vi "CNC-SpikePrime.vi"() -> ()   [LabVIEW 2020]
uses:
  Subs/ColorText/Code.xctl
panel:
  out "Array":dbl[][](array[numeric]) format="%#.2f"
  out "Bounds":T1 {"F Max" format="%#.1f"; "F Min" format="%#.1f"; "Z Max" format="%#.1f"; "Z Min" format="%#.1f"; "Y Max" format="%#.1f"; "Y Min" format="%#.1f"; "X Max" format="%#.1f"; "X Min" format="%#.1f"}
  out "Code":string(xcontrol)="import os\n\nfor i in range(10):\n     print(i)\n"
  in  "file (use dialog)":path=path "/Users/crogers/Downloads/PiMount_2.gcode"
  out "text":string="$X\nG21\nG90\nM6 T1\nG0 Z1.0 F300\nG0 X82.55 Y117.475 F6000\nG1 Z-2.2758 F250\nG1 Y123.825 F1000\nG1 X171.45\nG1 Y117.475\nG1 X82.55\nG1 X79.375 Y114.3\nG1 Y127.0\nG1 X174.625\nG1 Y114.3\nG1 X79.375\nG1 X76.2 Y111.125\nG1 Y130.175\nG1 X177.8\nG1 Y111.125\nG1 X76.2\nG1 X73.025 Y107.95\nG1 Y133.35\nG1 X180.975\nG1 Y107.95\nG1 X73.025\nG1 X69.85 Y104.775\nG1 Y136.525\nG1 X184.15\nG1 Y104.775\nG1 X69.85\nG1 X66.675 Y101.6\nG1 Y139.7\nG1 X187.325\nG1 Y101.6\nG1 X66.675\nG1 X63.5 Y98.425\nG1 Y142.875\nG1 X190.5\nG1 Y98.425\nG1 X63.5\nG1 X60.325 Y95.25\nG1 Y146.05\nG1 X193.675\nG1 Y95.25\nG1 X60.325\nG1 X57.15 Y92.075\nG1 Y149.225\nG1 X196.85\nG1 Y92.075\nG1 X57.15\nG1 X53.975 Y88.9\nG1 Y152.4\nG1 X200.025\nG1 Y88.9\nG1 X53.975\nG1 X50.8 Y85.725\nG1 Y155.575\nG1 X203.2\nG1 Y85.725\nG1 X50.8\nG1 X47.625 Y82.55\nG1 Y158.75\nG1 X206.375\nG1 Y82.55\nG1 X47.625\nG1 X44.45 Y79.375\nG1 Y161.925\nG1 X209.55\nG1 Y79.375\nG1 X44.45\nG1 X41.275 Y76.2\nG1 Y165.1\nG1 X212.725\nG1 Y76.2\nG1 X41.275\nG1 X38.1 Y73.025\nG1 Y168.275\nG1 X215.9\nG1 Y73.025\nG1 X38.1\nG1 X34.925 Y69.85\nG1 Y171.45\nG1 X219.075\nG1 Y69.85\nG1 X34.925\nG1 X31.8279 Y66.675\nG1 X31.7536 Y66.6787\nG1 X31.75 Y66.7528\nG1 Y174.5472\nG1 X31.7536 Y174.6214\nG1 X31.8279 Y174.625\nG1 X222.1721\nG1 X222.2464 Y174.6214\nG1 X222.25 Y174.5472\nG1 Y66.7528\nG1 X222.2464 Y66.6787\nG1 X222.1721 Y66.675\nG1 X31.8279\nG0 Z1.0 F300\nG0 X82.55 Y117.475 F6000\nG1 Z-4.2113 F250\nG1 Y123.825 F1000\nG1 X171.45\nG1 Y117.475\nG1 X82.55\nG1 X79.375 Y114.3\nG1 Y127.0\nG1 X174.625\nG1 Y114.3\nG1 X79.375\nG1 X76.2 Y111.125\nG1 Y130.175\nG1 X177.8\nG1 Y111.125\nG1 X76.2\nG1 X73.025 Y107.95\nG1 Y133.35\nG1 X180.975\nG1 Y107.95\nG1 X73.025\nG1 X69.85 Y104.775\nG1 Y136.525\nG1 X184.15\nG1 Y104.775\nG1 X69.85\nG1 X66.675 Y101.6\nG1 Y139.7\nG1 X187.325\nG1 Y101.6\nG1 X66.675\nG1 X63.5 Y98.425\nG1 Y142.875\nG1 X190.5\nG1 Y98.425\nG1 X63.5\nG1 X60.325 Y95.25\nG1 Y146.05\nG1 X193.675\nG1 Y95.25\nG1 X60.325\nG1 X57.15 Y92.075\nG1 Y149.225\nG1 X196.85\nG1 Y92.075\nG1 X57.15\nG1 X53.975 Y88.9\nG1 Y152.4\nG1 X200.025\nG1 Y88.9\nG1 X53.975\nG1 X50.8 Y85.725\nG1 Y155.575\nG1 X203.2\nG1 Y85.725\nG1 X50.8\nG1 X47.625 Y82.55\nG1 Y158.75\nG1 X206.375\nG1 Y82.55\nG1 X47.625\nG1 X44.45 Y79.375\nG1 Y161.925\nG1 X209.55\nG1 Y79.375\nG1 X44.45\nG1 X41.275 Y76.2\nG1 Y165.1\nG1 X212.725\nG1 Y76.2\nG1 X41.275\nG1 X38.1 Y73.025\nG1 Y168.275\nG1 X215.9\nG1 Y73.025\nG1 X38.1\nG1 X34.925 Y69.85\nG1 Y171.45\nG1 X219.075\nG1 Y69.85\nG1 X34.925\nG1 X31.8279 Y66.675\nG1 X31.7536 Y66.6787\nG1 X31.75 Y66.7528\nG1 Y174.5472\nG1 X31.7536 Y174.6214\nG1 X31.8279 Y174.625\nG1 X222.1721\nG1 X222.2464 Y174.6214\nG1 X222.25 Y174.5472\nG1 Y66.7528\nG1 X222.2464 Y66.6787\nG1 X222.1721 Y66.675\nG1 X31.8279\nG0 Z1.0 F300\nG0 X82.55 Y117.475 F6000\nG1 Z-6.35 F250\nG1 Y123.825 F1000\nG1 X171.45\nG1 Y117.475\nG1 X82.55\nG1 X79.375 Y114.3\nG1 Y127.0\nG1 X174.625\nG1 Y114.3\nG1 X79.375\nG1 X76.2 Y111.125\nG1 Y130.175\nG1 X177.8\nG1 Y111.125\nG1 X76.2\nG1 X73.025 Y107.95\nG1 Y133.35\nG1 X180.975\nG1 Y107.95\nG1 X73.025\nG1 X69.85 Y104.775\nG1 Y136.525\nG1 X184.15\nG1 Y104.775\nG1 X69.85\nG1 X66.675 Y101.6\nG1 Y139.7\nG1 X187.325\nG1 Y101.6\nG1 X66.675\nG1 X63.5 Y98.425\nG1 Y142.875\nG1 X190.5\nG1 Y98.425\nG1 X63.5\nG1 X60.325 Y95.25\nG1 Y146.05\nG1 X193.675\nG1 Y95.25\nG1 X60.325\nG1 X57.15 Y92.075\nG1 Y149.225\nG1 X196.85\nG1 Y92.075\nG1 X57.15\nG1 X53.975 Y88.9\nG1 Y152.4\nG1 X200.025\nG1 Y88.9\nG1 X53.975\nG1 X50.8 Y85.725\nG1 Y155.575\nG1 X203.2\nG1 Y85.725\nG1 X50.8\nG1 X47.625 Y82.55\nG1 Y158.75\nG1 X206.375\nG1 Y82.55\nG1 X47.625\nG1 X44.45 Y79.375\nG1 Y161.925\nG1 X209.55\nG1 Y79.375\nG1 X44.45\nG1 X41.275 Y76.2\nG1 Y165.1\nG1 X212.725\nG1 Y76.2\nG1 X41.275\nG1 X38.1 Y73.025\nG1 Y168.275\nG1 X215.9\nG1 Y73.025\nG1 X38.1\nG1 X34.925 Y69.85\nG1 Y171.45\nG1 X219.075\nG1 Y69.85\nG1 X34.925\nG1 X31.8279 Y66.675\nG1 X31.7536 Y66.6787\nG1 X31.75 Y66.7528\nG1 Y174.5472\nG1 X31.7536 Y174.6214\nG1 X31.8279 Y174.625\nG1 X222.1721\nG1 X222.2464 Y174.6214\nG1 X222.25 Y174.5472\nG1 Y66.7528\nG1 X222.2464 Y66.6787\nG1 X222.1721 Y66.675\nG1 X31.8279\nG0 Z1.0 F300\nG0 X104.775 Y117.475 F6000\nG1 Z-8.0823 F250\nG1 Y123.825 F1000\nG1 X149.225\nG1 Y117.475\nG1 X104.775\nG1 X101.6 Y114.3\nG1 Y127.0\nG1 X152.4\nG1 Y114.3\nG1 X101.6\nG1 X98.425 Y111.125\nG1 Y130.175\nG1 X155.575\nG1 Y111.125\nG1 X98.425\nG1 X95.25 Y107.95\nG1 Y133.35\nG1 X158.75\nG1 Y107.95\nG1 X95.25\nG1 X92.075 Y104.775\nG1 Y136.525\nG1 X161.925\nG1 Y104.775\nG1 X92.075\nG1 X88.9 Y101.6\nG1 Y139.7\nG1 X165.1\nG1 Y101.6\nG1 X88.9\nG1 X85.725 Y98.425\nG1 Y142.875\nG1 X168.275\nG1 Y98.425\nG1 X85.725\nG1 X82.55 Y95.25\nG1 Y146.05\nG1 X171.45\nG1 Y95.25\nG1 X82.55\nG1 X79.375 Y92.075\nG1 Y149.225\nG1 X174.625\nG1 Y92.075\nG1 X79.375\nG1 X76.2 Y88.9\nG1 Y152.4\nG1 X177.8\nG1 Y88.9\nG1 X76.2\nG1 X73.025 Y85.725\nG1 Y155.575\nG1 X180.975\nG1 Y85.725\nG1 X73.025\nG1 X69.85 Y82.55\nG1 Y158.75\nG1 X184.15\nG1 Y82.55\nG1 X69.85\nG1 X66.675 Y79.453\nG1 Y161.847\nG1 X66.6787 Y161.9214\nG1 X66.7528 Y161.925\nG1 X187.2472\nG1 X187.3214 Y161.9214\nG1 X187.325 Y161.847\nG1 Y79.453\nG1 X187.3214 Y79.3787\nG1 X187.2472 Y79.375\nG1 X66.7528\nG1 X66.6787 Y79.3787\nG1 X66.675 Y79.453\nG0 Z1.0 F300\nG0 X104.775 Y117.475 F6000\nG1 Z-10.0177 F250\nG1 Y123.825 F1000\nG1 X149.225\nG1 Y117.475\nG1 X104.775\nG1 X101.6 Y114.3\nG1 Y127.0\nG1 X152.4\nG1 Y114.3\nG1 X101.6\nG1 X98.425 Y111.125\nG1 Y130.175\nG1 X155.575\nG1 Y111.125\nG1 X98.425\nG1 X95.25 Y107.95\nG1 Y133.35\nG1 X158.75\nG1 Y107.95\nG1 X95.25\nG1 X92.075 Y104.775\nG1 Y136.525\nG1 X161.925\nG1 Y104.775\nG1 X92.075\nG1 X88.9 Y101.6\nG1 Y139.7\nG1 X165.1\nG1 Y101.6\nG1 X88.9\nG1 X85.725 Y98.425\nG1 Y142.875\nG1 X168.275\nG1 Y98.425\nG1 X85.725\nG1 X82.55 Y95.25\nG1 Y146.05\nG1 X171.45\nG1 Y95.25\nG1 X82.55\nG1 X79.375 Y92.075\nG1 Y149.225\nG1 X174.625\nG1 Y92.075\nG1 X79.375\nG1 X76.2 Y88.9\nG1 Y152.4\nG1 X177.8\nG1 Y88.9\nG1 X76.2\nG1 X73.025 Y85.725\nG1 Y155.575\nG1 X180.975\nG1 Y85.725\nG1 X73.025\nG1 X69.85 Y82.55\nG1 Y158.75\nG1 X184.15\nG1 Y82.55\nG1 X69.85\nG1 X66.675 Y79.453\nG1 Y161.847\nG1 X66.6787 Y161.9214\nG1 X66.7528 Y161.925\nG1 X187.2472\nG1 X187.3214 Y161.9214\nG1 X187.325 Y161.847\nG1 Y79.453\nG1 X187.3214 Y79.3787\nG1 X187.2472 Y79.375\nG1 X66.7528\nG1 X66.6787 Y79.3787\nG1 X66.675 Y79.453\nG0 Z1.0 F300\nG0 X104.775 Y117.475 F6000\nG1 Z-11.9532 F250\nG1 Y123.825 F1000\nG1 X149.225\nG1 Y117.475\nG1 X104.775\nG1 X101.6 Y114.3\nG1 Y127.0\nG1 X152.4\nG1 Y114.3\nG1 X101.6\nG1 X98.425 Y111.125\nG1 Y130.175\nG1 X155.575\nG1 Y111.125\nG1 X98.425\nG1 X95.25 Y107.95\nG1 Y133.35\nG1 X158.75\nG1 Y107.95\nG1 X95.25\nG1 X92.075 Y104.775\nG1 Y136.525\nG1 X161.925\nG1 Y104.775\nG1 X92.075\nG1 X88.9 Y101.6\nG1 Y139.7\nG1 X165.1\nG1 Y101.6\nG1 X88.9\nG1 X85.725 Y98.425\nG1 Y142.875\nG1 X168.275\nG1 Y98.425\nG1 X85.725\nG1 X82.55 Y95.25\nG1 Y146.05\nG1 X171.45\nG1 Y95.25\nG1 X82.55\nG1 X79.375 Y92.075\nG1 Y149.225\nG1 X174.625\nG1 Y92.075\nG1 X79.375\nG1 X76.2 Y88.9\nG1 Y152.4\nG1 X177.8\nG1 Y88.9\nG1 X76.2\nG1 X73.025 Y85.725\nG1 Y155.575\nG1 X180.975\nG1 Y85.725\nG1 X73.025\nG1 X69.85 Y82.55\nG1 Y158.75\nG1 X184.15\nG1 Y82.55\nG1 X69.85\nG1 X66.675 Y79.453\nG1 Y161.847\nG1 X66.6787 Y161.9214\nG1 X66.7528 Y161.925\nG1 X187.2472\nG1 X187.3214 Y161.9214\nG1 X187.325 Y161.847\nG1 Y79.453\nG1 X187.3214 Y79.3787\nG1 X187.2472 Y79.375\nG1 X66.7528\nG1 X66.6787 Y79.3787\nG1 X66.675 Y79.453\nG0 Z1.0 F300\nG0 X104.775 Y117.475 F6000\nG1 Z-13.8887 F250\nG1 Y123.825 F1000\nG1 X149.225\nG1 Y117.475\nG1 X104.775\nG1 X101.6 Y114.3\nG1 Y127.0\nG1 X152.4\nG1 Y114.3\nG1 X101.6\nG1 X98.425 Y111.125\nG1 Y130.175\nG1 X155.575\nG1 Y111.125\nG1 X98.425\nG1 X95.25 Y107.95\nG1 Y133.35\nG1 X158.75\nG1 Y107.95\nG1 X95.25\nG1 X92.075 Y104.775\nG1 Y136.525\nG1 X161.925\nG1 Y104.775\nG1 X92.075\nG1 X88.9 Y101.6\nG1 Y139.7\nG1 X165.1\nG1 Y101.6\nG1 X88.9\nG1 X85.725 Y98.425\nG1 Y142.875\nG1 X168.275\nG1 Y98.425\nG1 X85.725\nG1 X82.55 Y95.25\nG1 Y146.05\nG1 X171.45\nG1 Y95.25\nG1 X82.55\nG1 X79.375 Y92.075\nG1 Y149.225\nG1 X174.625\nG1 Y92.075\nG1 X79.375\nG1 X76.2 Y88.9\nG1 Y152.4\nG1 X177.8\nG1 Y88.9\nG1 X76.2\nG1 X73.025 Y85.725\nG1 Y155.575\nG1 X180.975\nG1 Y85.725\nG1 X73.025\nG1 X69.85 Y82.55\nG1 Y158.75\nG1 X184.15\nG1 Y82.55\nG1 X69.85\nG1 X66.675 Y79.453\nG1 Y161.847\nG1 X66.6787 Y161.9214\nG1 X66.7528 Y161.925\nG1 X187.2472\nG1 X187.3214 Y161.9214\nG1 X187.325 Y161.847\nG1 Y79.453\nG1 X187.3214 Y79.3787\nG1 X187.2472 Y79.375\nG1 X66.7528\nG1 X66.6787 Y79.3787\nG1 X66.675 Y79.453\nG0 Z1.0 F300\nG0 X104.775 Y117.475 F6000\nG1 Z-15.179 F250\nG1 Y123.825 F1000\nG1 X149.225\nG1 Y117.475\nG1 X104.775\nG1 X101.6 Y114.3\nG1 Y127.0\nG1 X152.4\nG1 Y114.3\nG1 X101.6\nG1 X98.425 Y111.125\nG1 Y130.175\nG1 X155.575\nG1 Y111.125\nG1 X98.425\nG1 X95.25 Y107.95\nG1 Y133.35\nG1 X158.75\nG1 Y107.95\nG1 X95.25\nG1 X92.075 Y104.775\nG1 Y136.525\nG1 X161.925\nG1 Y104.775\nG1 X92.075\nG1 X88.9 Y101.6\nG1 Y139.7\nG1 X165.1\nG1 Y101.6\nG1 X88.9\nG1 X85.725 Y98.425\nG1 Y142.875\nG1 X168.275\nG1 Y98.425\nG1 X85.725\nG1 X82.55 Y95.25\nG1 Y146.05\nG1 X171.45\nG1 Y95.25\nG1 X82.55\nG1 X79.375 Y92.075\nG1 Y149.225\nG1 X174.625\nG1 Y92.075\nG1 X79.375\nG1 X76.2 Y88.9\nG1 Y152.4\nG1 X177.8\nG1 Y88.9\nG1 X76.2\nG1 X73.025 Y85.725\nG1 Y155.575\nG1 X180.975\nG1 Y85.725\nG1 X73.025\nG1 X69.85 Y82.55\nG1 Y158.75\nG1 X184.15\nG1 Y82.55\nG1 X69.85\nG1 X66.675 Y79.453\nG1 Y161.847\nG1 X66.6787 Y161.9214\nG1 X66.7528 Y161.925\nG1 X187.2472\nG1 X187.3214 Y161.9214\nG1 X187.325 Y161.847\nG1 Y79.453\nG1 X187.3214 Y79.3787\nG1 X187.2472 Y79.375\nG1 X66.7528\nG1 X66.6787 Y79.3787\nG1 X66.675 Y79.453\nG0 Z1.0 F300\nG0 X104.775 Y117.475 F6000\nG1 Z-17.1145 F250\nG1 Y123.825 F1000\nG1 X149.225\nG1 Y117.475\nG1 X104.775\nG1 X101.6 Y114.3\nG1 Y127.0\nG1 X152.4\nG1 Y114.3\nG1 X101.6\nG1 X98.425 Y111.125\nG1 Y130.175\nG1 X155.575\nG1 Y111.125\nG1 X98.425\nG1 X95.25 Y107.95\nG1 Y133.35\nG1 X158.75\nG1 Y107.95\nG1 X95.25\nG1 X92.075 Y104.775\nG1 Y136.525\nG1 X161.925\nG1 Y104.775\nG1 X92.075\nG1 X88.9 Y101.6\nG1 Y139.7\nG1 X165.1\nG1 Y101.6\nG1 X88.9\nG1 X85.725 Y98.425\nG1 Y142.875\nG1 X168.275\nG1 Y98.425\nG1 X85.725\nG1 X82.55 Y95.25\nG1 Y146.05\nG1 X171.45\nG1 Y95.25\nG1 X82.55\nG1 X79.375 Y92.075\nG1 Y149.225\nG1 X174.625\nG1 Y92.075\nG1 X79.375\nG1 X76.2 Y88.9\nG1 Y152.4\nG1 X177.8\nG1 Y88.9\nG1 X76.2\nG1 X73.025 Y85.725\nG1 Y155.575\nG1 X180.975\nG1 Y85.725\nG1 X73.025\nG1 X69.85 Y82.55\nG1 Y158.75\nG1 X184.15\nG1 Y82.55\nG1 X69.85\nG1 X66.675 Y79.453\nG1 Y161.847\nG1 X66.6787 Y161.9214\nG1 X66.7528 Y161.925\nG1 X187.2472\nG1 X187.3214 Y161.9214\nG1 X187.325 Y161.847\nG1 Y79.453\nG1 X187.3214 Y79.3787\nG1 X187.2472 Y79.375\nG1 X66.7528\nG1 X66.6787 Y79.3787\nG1 X66.675 Y79.453\nG0 Z1.0 F300\nG0 X104.775 Y117.475 F6000\nG1 Z-19.05 F250\nG1 Y123.825 F1000\nG1 X149.225\nG1 Y117.475\nG1 X104.775\nG1 X101.6 Y114.3\nG1 Y127.0\nG1 X152.4\nG1 Y114.3\nG1 X101.6\nG1 X98.425 Y111.125\nG1 Y130.175\nG1 X155.575\nG1 Y111.125\nG1 X98.425\nG1 X95.25 Y107.95\nG1 Y133.35\nG1 X158.75\nG1 Y107.95\nG1 X95.25\nG1 X92.075 Y104.775\nG1 Y136.525\nG1 X161.925\nG1 Y104.775\nG1 X92.075\nG1 X88.9 Y101.6\nG1 Y139.7\nG1 X165.1\nG1 Y101.6\nG1 X88.9\nG1 X85.725 Y98.425\nG1 Y142.875\nG1 X168.275\nG1 Y98.425\nG1 X85.725\nG1 X82.55 Y95.25\nG1 Y146.05\nG1 X171.45\nG1 Y95.25\nG1 X82.55\nG1 X79.375 Y92.075\nG1 Y149.225\nG1 X174.625\nG1 Y92.075\nG1 X79.375\nG1 X76.2 Y88.9\nG1 Y152.4\nG1 X177.8\nG1 Y88.9\nG1 X76.2\nG1 X73.025 Y85.725\nG1 Y155.575\nG1 X180.975\nG1 Y85.725\nG1 X73.025\nG1 X69.85 Y82.55\nG1 Y158.75\nG1 X184.15\nG1 Y82.55\nG1 X69.85\nG1 X66.675 Y79.453\nG1 Y161.847\nG1 X66.6787 Y161.9214\nG1 X66.7528 Y161.925\nG1 X187.2471\nG1 X187.3214 Y161.9214\nG1 X187.325 Y161.847\nG1 Y79.453\nG1 X187.3214 Y79.3787\nG1 X187.2472 Y79.375\nG1 X66.7529\nG1 X66.6787 Y79.3787\nG1 X66.675 Y79.453\nG0 Z1.0 F300\nG0 X12.6221 Y47.625 F6000\nG1 Z-2.2758 F300\nG1 X11.1436 Y47.6976 F1000\nG1 X9.6022 Y47.9263\nG1 X8.0906 Y48.3049\nG1 X6.6235 Y48.8299\nG1 X5.2148 Y49.4961\nG1 X3.8782 Y50.2972\nG1 X2.6266 Y51.2255\nG1 X1.472 Y52.272\nG1 X0.4255 Y53.4266\nG1 X-0.5028 Y54.6782\nG1 X-1.3039 Y56.0148\nG1 X-1.9701 Y57.4234\nG1 X-2.4951 Y58.8906\nG1 X-2.8737 Y60.4022\nG1 X-3.1024 Y61.9436\nG1 X-3.175 Y63.4221\nG1 Y177.8779\nG1 X-3.1024 Y179.3564\nG1 X-2.8737 Y180.8978\nG1 X-2.4951 Y182.4094\nG1 X-1.9701 Y183.8766\nG1 X-1.3039 Y185.2853\nG1 X-0.5028 Y186.6218\nG1 X0.4255 Y187.8734\nG1 X1.472 Y189.028\nG1 X2.6266 Y190.0745\nG1 X3.8782 Y191.0028\nG1 X5.2148 Y191.8039\nG1 X6.6235 Y192.4701\nG1 X8.0906 Y192.9951\nG1 X9.6022 Y193.3737\nG1 X11.1436 Y193.6024\nG1 X12.6221 Y193.675\nG1 X190.4222\nG1 X191.4332 Y193.7247\nG1 X192.3575 Y193.8618\nG1 X193.2639 Y194.0888\nG1 X194.1436 Y194.4036\nG1 X194.9882 Y194.8031\nG1 X195.7896 Y195.2834\nG1 X196.5401 Y195.84\nG1 X197.2325 Y196.4675\nG1 X197.86 Y197.1598\nG1 X198.4166 Y197.9103\nG1 X198.8969 Y198.7117\nG1 X199.2964 Y199.5564\nG1 X199.6112 Y200.4362\nG1 X199.8382 Y201.3426\nG1 X199.9753 Y202.2668\nG1 X200.025 Y203.278\nG1 Y228.6779\nG1 X200.0976 Y230.1564\nG1 X200.3263 Y231.6978\nG1 X200.7049 Y233.2094\nG1 X201.2299 Y234.6766\nG1 X201.8961 Y236.0852\nG1 X202.6972 Y237.4218\nG1 X203.6255 Y238.6734\nG1 X204.672 Y239.828\nG1 X205.8266 Y240.8745\nG1 X207.0782 Y241.8028\nG1 X208.4148 Y242.6039\nG1 X209.8234 Y243.2701\nG1 X211.2906 Y243.7951\nG1 X212.8022 Y244.1737\nG1 X214.3436 Y244.4024\nG1 X215.8221 Y244.475\nG1 X257.175\nG1 Y-3.175\nG1 X215.8221\nG1 X214.3436 Y-3.1024\nG1 X212.8022 Y-2.8737\nG1 X211.2906 Y-2.4951\nG1 X209.8234 Y-1.9701\nG1 X208.4148 Y-1.3039\nG1 X207.0782 Y-0.5028\nG1 X205.8266 Y0.4255\nG1 X204.672 Y1.472\nG1 X203.6255 Y2.6266\nG1 X202.6972 Y3.8782\nG1 X201.8961 Y5.2148\nG1 X201.2299 Y6.6234\nG1 X200.7049 Y8.0906\nG1 X200.3263 Y9.6022\nG1 X200.0976 Y11.1436\nG1 X200.025 Y12.6221\nG1 Y38.022\nG1 X199.9753 Y39.0332\nG1 X199.8382 Y39.9574\nG1 X199.6112 Y40.8638\nG1 X199.2964 Y41.7436\nG1 X198.8969 Y42.5883\nG1 X198.4166 Y43.3897\nG1 X197.86 Y44.1402\nG1 X197.2325 Y44.8325\nG1 X196.5401 Y45.46\nG1 X195.7896 Y46.0166\nG1 X194.9882 Y46.4969\nG1 X194.1436 Y46.8964\nG1 X193.2639 Y47.2112\nG1 X192.3575 Y47.4382\nG1 X191.4332 Y47.5753\nG1 X190.4222 Y47.625\nG1 X12.6221\nG1 Z-4.2113 F250\nG1 X11.1436 Y47.6976 F1000\nG1 X9.6022 Y47.9263\nG1 X8.0906 Y48.3049\nG1 X6.6235 Y48.8299\nG1 X5.2148 Y49.4961\nG1 X3.8782 Y50.2972\nG1 X2.6266 Y51.2255\nG1 X1.472 Y52.272\nG1 X0.4255 Y53.4266\nG1 X-0.5028 Y54.6782\nG1 X-1.3039 Y56.0148\nG1 X-1.9701 Y57.4234\nG1 X-2.4951 Y58.8906\nG1 X-2.8737 Y60.4022\nG1 X-3.1024 Y61.9436\nG1 X-3.175 Y63.4221\nG1 Y177.8779\nG1 X-3.1024 Y179.3564\nG1 X-2.8737 Y180.8978\nG1 X-2.4951 Y182.4094\nG1 X-1.9701 Y183.8766\nG1 X-1.3039 Y185.2853\nG1 X-0.5028 Y186.6218\nG1 X0.4255 Y187.8734\nG1 X1.472 Y189.028\nG1 X2.6266 Y190.0745\nG1 X3.8782 Y191.0028\nG1 X5.2148 Y191.8039\nG1 X6.6235 Y192.4701\nG1 X8.0906 Y192.9951\nG1 X9.6022 Y193.3737\nG1 X11.1436 Y193.6024\nG1 X12.6221 Y193.675\nG1 X190.4222\nG1 X191.4332 Y193.7247\nG1 X192.3575 Y193.8618\nG1 X193.2639 Y194.0888\nG1 X194.1436 Y194.4036\nG1 X194.9882 Y194.8031\nG1 X195.7896 Y195.2834\nG1 X196.5401 Y195.84\nG1 X197.2325 Y196.4675\nG1 X197.86 Y197.1598\nG1 X198.4166 Y197.9103\nG1 X198.8969 Y198.7117\nG1 X199.2964 Y199.5564\nG1 X199.6112 Y200.4362\nG1 X199.8382 Y201.3426\nG1 X199.9753 Y202.2668\nG1 X200.025 Y203.278\nG1 Y228.6779\nG1 X200.0976 Y230.1564\nG1 X200.3263 Y231.6978\nG1 X200.7049 Y233.2094\nG1 X201.2299 Y234.6766\nG1 X201.8961 Y236.0852\nG1 X202.6972 Y237.4218\nG1 X203.6255 Y238.6734\nG1 X204.672 Y239.828\nG1 X205.8266 Y240.8745\nG1 X207.0782 Y241.8028\nG1 X208.4148 Y242.6039\nG1 X209.8234 Y243.2701\nG1 X211.2906 Y243.7951\nG1 X212.8022 Y244.1737\nG1 X214.3436 Y244.4024\nG1 X215.8221 Y244.475\nG1 X257.175\nG1 Y-3.175\nG1 X215.8221\nG1 X214.3436 Y-3.1024\nG1 X212.8022 Y-2.8737\nG1 X211.2906 Y-2.4951\nG1 X209.8234 Y-1.9701\nG1 X208.4148 Y-1.3039\nG1 X207.0782 Y-0.5028\nG1 X205.8266 Y0.4255\nG1 X204.672 Y1.472\nG1 X203.6255 Y2.6266\nG1 X202.6972 Y3.8782\nG1 X201.8961 Y5.2148\nG1 X201.2299 Y6.6234\nG1 X200.7049 Y8.0906\nG1 X200.3263 Y9.6022\nG1 X200.0976 Y11.1436\nG1 X200.025 Y12.6221\nG1 Y38.022\nG1 X199.9753 Y39.0332\nG1 X199.8382 Y39.9574\nG1 X199.6112 Y40.8638\nG1 X199.2964 Y41.7436\nG1 X198.8969 Y42.5883\nG1 X198.4166 Y43.3897\nG1 X197.86 Y44.1402\nG1 X197.2325 Y44.8325\nG1 X196.5401 Y45.46\nG1 X195.7896 Y46.0166\nG1 X194.9882 Y46.4969\nG1 X194.1436 Y46.8964\nG1 X193.2639 Y47.2112\nG1 X192.3575 Y47.4382\nG1 X191.4332 Y47.5753\nG1 X190.4222 Y47.625\nG1 X12.6221\nG1 Z-6.35 F250\nG1 X11.1436 Y47.6976 F1000\nG1 X9.6022 Y47.9263\nG1 X8.0906 Y48.3049\nG1 X6.6235 Y48.8299\nG1 X5.2148 Y49.4961\nG1 X3.8782 Y50.2972\nG1 X2.6266 Y51.2255\nG1 X1.472 Y52.272\nG1 X0.4255 Y53.4266\nG1 X-0.5028 Y54.6782\nG1 X-1.3039 Y56.0148\nG1 X-1.9701 Y57.4234\nG1 X-2.4951 Y58.8906\nG1 X-2.8737 Y60.4022\nG1 X-3.1024 Y61.9436\nG1 X-3.175 Y63.4221\nG1 Y177.8779\nG1 X-3.1024 Y179.3564\nG1 X-2.8737 Y180.8978\nG1 X-2.4951 Y182.4094\nG1 X-1.9701 Y183.8766\nG1 X-1.3039 Y185.2853\nG1 X-0.5028 Y186.6218\nG1 X0.4255 Y187.8734\nG1 X1.472 Y189.028\nG1 X2.6266 Y190.0745\nG1 X3.8782 Y191.0028\nG1 X5.2148 Y191.8039\nG1 X6.6235 Y192.4701\nG1 X8.0906 Y192.9951\nG1 X9.6022 Y193.3737\nG1 X11.1436 Y193.6024\nG1 X12.6221 Y193.675\nG1 X190.4222\nG1 X191.4332 Y193.7247\nG1 X192.3575 Y193.8618\nG1 X193.2639 Y194.0888\nG1 X194.1436 Y194.4036\nG1 X194.9882 Y194.8031\nG1 X195.7896 Y195.2834\nG1 X196.5401 Y195.84\nG1 X197.2325 Y196.4675\nG1 X197.86 Y197.1598\nG1 X198.4166 Y197.9103\nG1 X198.8969 Y198.7117\nG1 X199.2964 Y199.5564\nG1 X199.6112 Y200.4362\nG1 X199.8382 Y201.3426\nG1 X199.9753 Y202.2668\nG1 X200.025 Y203.278\nG1 Y228.6779\nG1 X200.0976 Y230.1564\nG1 X200.3263 Y231.6978\nG1 X200.7049 Y233.2094\nG1 X201.2299 Y234.6766\nG1 X201.8961 Y236.0852\nG1 X202.6972 Y237.4218\nG1 X203.6255 Y238.6734\nG1 X204.672 Y239.828\nG1 X205.8266 Y240.8745\nG1 X207.0782 Y241.8028\nG1 X208.4148 Y242.6039\nG1 X209.8234 Y243.2701\nG1 X211.2906 Y243.7951\nG1 X212.8022 Y244.1737\nG1 X214.3436 Y244.4024\nG1 X215.8221 Y244.475\nG1 X257.175\nG1 Y-3.175\nG1 X215.8221\nG1 X214.3436 Y-3.1024\nG1 X212.8022 Y-2.8737\nG1 X211.2906 Y-2.4951\nG1 X209.8234 Y-1.9701\nG1 X208.4148 Y-1.3039\nG1 X207.0782 Y-0.5028\nG1 X205.8266 Y0.4255\nG1 X204.672 Y1.472\nG1 X203.6255 Y2.6266\nG1 X202.6972 Y3.8782\nG1 X201.8961 Y5.2148\nG1 X201.2299 Y6.6234\nG1 X200.7049 Y8.0906\nG1 X200.3263 Y9.6022\nG1 X200.0976 Y11.1436\nG1 X200.025 Y12.6221\nG1 Y38.022\nG1 X199.9753 Y39.0332\nG1 X199.8382 Y39.9574\nG1 X199.6112 Y40.8638\nG1 X199.2964 Y41.7436\nG1 X198.8969 Y42.5883\nG1 X198.4166 Y43.3897\nG1 X197.86 Y44.1402\nG1 X197.2325 Y44.8325\nG1 X196.5401 Y45.46\nG1 X195.7896 Y46.0166\nG1 X194.9882 Y46.4969\nG1 X194.1436 Y46.8964\nG1 X193.2639 Y47.2112\nG1 X192.3575 Y47.4382\nG1 X191.4332 Y47.5753\nG1 X190.4222 Y47.625\nG1 X12.6221\nG1 Z-8.0823 F250\nG1 X11.1436 Y47.6976 F1000\nG1 X9.6022 Y47.9263\nG1 X8.0906 Y48.3049\nG1 X6.6235 Y48.8299\nG1 X5.2148 Y49.4961\nG1 X3.8782 Y50.2972\nG1 X2.6266 Y51.2255\nG1 X1.472 Y52.272\nG1 X0.4255 Y53.4266\nG1 X-0.5028 Y54.6782\nG1 X-1.3039 Y56.0148\nG1 X-1.9701 Y57.4234\nG1 X-2.4951 Y58.8906\nG1 X-2.8737 Y60.4022\nG1 X-3.1024 Y61.9436\nG1 X-3.175 Y63.4221\nG1 Y177.8779\nG1 X-3.1024 Y179.3564\nG1 X-2.8737 Y180.8978\nG1 X-2.4951 Y182.4094\nG1 X-1.9701 Y183.8766\nG1 X-1.3039 Y185.2853\nG1 X-0.5028 Y186.6218\nG1 X0.4255 Y187.8734\nG1 X1.472 Y189.028\nG1 X2.6266 Y190.0745\nG1 X3.8782 Y191.0028\nG1 X5.2148 Y191.8039\nG1 X6.6235 Y192.4701\nG1 X8.0906 Y192.9951\nG1 X9.6022 Y193.3737\nG1 X11.1436 Y193.6024\nG1 X12.6221 Y193.675\nG1 X190.4222\nG1 X191.4332 Y193.7247\nG1 X192.3575 Y193.8618\nG1 X193.2639 Y194.0888\nG1 X194.1436 Y194.4036\nG1 X194.9882 Y194.8031\nG1 X195.7896 Y195.2834\nG1 X196.5401 Y195.84\nG1 X197.2325 Y196.4675\nG1 X197.86 Y197.1598\nG1 X198.4166 Y197.9103\nG1 X198.8969 Y198.7117\nG1 X199.2964 Y199.5564\nG1 X199.6112 Y200.4362\nG1 X199.8382 Y201.3426\nG1 X199.9753 Y202.2668\nG1 X200.025 Y203.278\nG1 Y228.6779\nG1 X200.0976 Y230.1564\nG1 X200.3263 Y231.6978\nG1 X200.7049 Y233.2094\nG1 X201.2299 Y234.6766\nG1 X201.8961 Y236.0852\nG1 X202.6972 Y237.4218\nG1 X203.6255 Y238.6734\nG1 X204.672 Y239.828\nG1 X205.8266 Y240.8745\nG1 X207.0782 Y241.8028\nG1 X208.4148 Y242.6039\nG1 X209.8234 Y243.2701\nG1 X211.2906 Y243.7951\nG1 X212.8022 Y244.1737\nG1 X214.3436 Y244.4024\nG1 X215.8221 Y244.475\nG1 X257.175\nG1 Y-3.175\nG1 X215.8221\nG1 X214.3436 Y-3.1024\nG1 X212.8022 Y-2.8737\nG1 X211.2906 Y-2.4951\nG1 X209.8234 Y-1.9701\nG1 X208.4148 Y-1.3039\nG1 X207.0782 Y-0.5028\nG1 X205.8266 Y0.4255\nG1 X204.672 Y1.472\nG1 X203.6255 Y2.6266\nG1 X202.6972 Y3.8782\nG1 X201.8961 Y5.2148\nG1 X201.2299 Y6.6234\nG1 X200.7049 Y8.0906\nG1 X200.3263 Y9.6022\nG1 X200.0976 Y11.1436\nG1 X200.025 Y12.6221\nG1 Y38.022\nG1 X199.9753 Y39.0332\nG1 X199.8382 Y39.9574\nG1 X199.6112 Y40.8638\nG1 X199.2964 Y41.7436\nG1 X198.8969 Y42.5883\nG1 X198.4166 Y43.3897\nG1 X197.86 Y44.1402\nG1 X197.2325 Y44.8325\nG1 X196.5401 Y45.46\nG1 X195.7896 Y46.0166\nG1 X194.9882 Y46.4969\nG1 X194.1436 Y46.8964\nG1 X193.2639 Y47.2112\nG1 X192.3575 Y47.4382\nG1 X191.4332 Y47.5753\nG1 X190.4222 Y47.625\nG1 X12.6221\nG1 Z-10.0177 F250\nG1 X11.1436 Y47.6976 F1000\nG1 X9.6022 Y47.9263\nG1 X8.0906 Y48.3049\nG1 X6.6235 Y48.8299\nG1 X5.2148 Y49.4961\nG1 X3.8782 Y50.2972\nG1 X2.6266 Y51.2255\nG1 X1.472 Y52.272\nG1 X0.4255 Y53.4266\nG1 X-0.5028 Y54.6782\nG1 X-1.3039 Y56.0148\nG1 X-1.9701 Y57.4234\nG1 X-2.4951 Y58.8906\nG1 X-2.8737 Y60.4022\nG1 X-3.1024 Y61.9436\nG1 X-3.175 Y63.4221\nG1 Y177.8779\nG1 X-3.1024 Y179.3564\nG1 X-2.8737 Y180.8978\nG1 X-2.4951 Y182.4094\nG1 X-1.9701 Y183.8766\nG1 X-1.3039 Y185.2853\nG1 X-0.5028 Y186.6218\nG1 X0.4255 Y187.8734\nG1 X1.472 Y189.028\nG1 X2.6266 Y190.0745\nG1 X3.8782 Y191.0028\nG1 X5.2148 Y191.8039\nG1 X6.6235 Y192.4701\nG1 X8.0906 Y192.9951\nG1 X9.6022 Y193.3737\nG1 X11.1436 Y193.6024\nG1 X12.6221 Y193.675\nG1 X190.4222\nG1 X191.4332 Y193.7247\nG1 X192.3575 Y193.8618\nG1 X193.2639 Y194.0888\nG1 X194.1436 Y194.4036\nG1 X194.9882 Y194.8031\nG1 X195.7896 Y195.2834\nG1 X196.5401 Y195.84\nG1 X197.2325 Y196.4675\nG1 X197.86 Y197.1598\nG1 X198.4166 Y197.9103\nG1 X198.8969 Y198.7117\nG1 X199.2964 Y199.5564\nG1 X199.6112 Y200.4362\nG1 X199.8382 Y201.3426\nG1 X199.9753 Y202.2668\nG1 X200.025 Y203.278\nG1 Y228.6779\nG1 X200.0976 Y230.1564\nG1 X200.3263 Y231.6978\nG1 X200.7049 Y233.2094\nG1 X201.2299 Y234.6766\nG1 X201.8961 Y236.0852\nG1 X202.6972 Y237.4218\nG1 X203.6255 Y238.6734\nG1 X204.672 Y239.828\nG1 X205.8266 Y240.8745\nG1 X207.0782 Y241.8028\nG1 X208.4148 Y242.6039\nG1 X209.8234 Y243.2701\nG1 X211.2906 Y243.7951\nG1 X212.8022 Y244.1737\nG1 X214.3436 Y244.4024\nG1 X215.8221 Y244.475\nG1 X257.175\nG1 Y-3.175\nG1 X215.8221\nG1 X214.3436 Y-3.1024\nG1 X212.8022 Y-2.8737\nG1 X211.2906 Y-2.4951\nG1 X209.8234 Y-1.9701\nG1 X208.4148 Y-1.3039\nG1 X207.0782 Y-0.5028\nG1 X205.8266 Y0.4255\nG1 X204.672 Y1.472\nG1 X203.6255 Y2.6266\nG1 X202.6972 Y3.8782\nG1 X201.8961 Y5.2148\nG1 X201.2299 Y6.6234\nG1 X200.7049 Y8.0906\nG1 X200.3263 Y9.6022\nG1 X200.0976 Y11.1436\nG1 X200.025 Y12.6221\nG1 Y38.022\nG1 X199.9753 Y39.0332\nG1 X199.8382 Y39.9574\nG1 X199.6112 Y40.8638\nG1 X199.2964 Y41.7436\nG1 X198.8969 Y42.5883\nG1 X198.4166 Y43.3897\nG1 X197.86 Y44.1402\nG1 X197.2325 Y44.8325\nG1 X196.5401 Y45.46\nG1 X195.7896 Y46.0166\nG1 X194.9882 Y46.4969\nG1 X194.1436 Y46.8964\nG1 X193.2639 Y47.2112\nG1 X192.3575 Y47.4382\nG1 X191.4332 Y47.5753\nG1 X190.4222 Y47.625\nG1 X12.6221\nG1 Z-11.9532 F250\nG1 X11.1436 Y47.6976 F1000\nG1 X9.6022 Y47.9263\nG1 X8.0906 Y48.3049\nG1 X6.6235 Y48.8299\nG1 X5.2148 Y49.4961\nG1 X3.8782 Y50.2972\nG1 X2.6266 Y51.2255\nG1 X1.472 Y52.272\nG1 X0.4255 Y53.4266\nG1 X-0.5028 Y54.6782\nG1 X-1.3039 Y56.0148\nG1 X-1.9701 Y57.4234\nG1 X-2.4951 Y58.8906\nG1 X-2.8737 Y60.4022\nG1 X-3.1024 Y61.9436\nG1 X-3.175 Y63.4221\nG1 Y177.8779\nG1 X-3.1024 Y179.3564\nG1 X-2.8737 Y180.8978\nG1 X-2.4951 Y182.4094\nG1 X-1.9701 Y183.8766\nG1 X-1.3039 Y185.2853\nG1 X-0.5028 Y186.6218\nG1 X0.4255 Y187.8734\nG1 X1.472 Y189.028\nG1 X2.6266 Y190.0745\nG1 X3.8782 Y191.0028\nG1 X5.2148 Y191.8039\nG1 X6.6235 Y192.4701\nG1 X8.0906 Y192.9951\nG1 X9.6022 Y193.3737\nG1 X11.1436 Y193.6024\nG1 X12.6221 Y193.675\nG1 X190.4222\nG1 X191.4332 Y193.7247\nG1 X192.3575 Y193.8618\nG1 X193.2639 Y194.0888\nG1 X194.1436 Y194.4036\nG1 X194.9882 Y194.8031\nG1 X195.7896 Y195.2834\nG1 X196.5401 Y195.84\nG1 X197.2325 Y196.4675\nG1 X197.86 Y197.1598\nG1 X198.4166 Y197.9103\nG1 X198.8969 Y198.7117\nG1 X199.2964 Y199.5564\nG1 X199.6112 Y200.4362\nG1 X199.8382 Y201.3426\nG1 X199.9753 Y202.2668\nG1 X200.025 Y203.278\nG1 Y228.6779\nG1 X200.0976 Y230.1564\nG1 X200.3263 Y231.6978\nG1 X200.7049 Y233.2094\nG1 X201.2299 Y234.6766\nG1 X201.8961 Y236.0852\nG1 X202.6972 Y237.4218\nG1 X203.6255 Y238.6734\nG1 X204.672 Y239.828\nG1 X205.8266 Y240.8745\nG1 X207.0782 Y241.8028\nG1 X208.4148 Y242.6039\nG1 X209.8234 Y243.2701\nG1 X211.2906 Y243.7951\nG1 X212.8022 Y244.1737\nG1 X214.3436 Y244.4024\nG1 X215.8221 Y244.475\nG1 X257.175\nG1 Y-3.175\nG1 X215.8221\nG1 X214.3436 Y-3.1024\nG1 X212.8022 Y-2.8737\nG1 X211.2906 Y-2.4951\nG1 X209.8234 Y-1.9701\nG1 X208.4148 Y-1.3039\nG1 X207.0782 Y-0.5028\nG1 X205.8266 Y0.4255\nG1 X204.672 Y1.472\nG1 X203.6255 Y2.6266\nG1 X202.6972 Y3.8782\nG1 X201.8961 Y5.2148\nG1 X201.2299 Y6.6234\nG1 X200.7049 Y8.0906\nG1 X200.3263 Y9.6022\nG1 X200.0976 Y11.1436\nG1 X200.025 Y12.6221\nG1 Y38.022\nG1 X199.9753 Y39.0332\nG1 X199.8382 Y39.9574\nG1 X199.6112 Y40.8638\nG1 X199.2964 Y41.7436\nG1 X198.8969 Y42.5883\nG1 X198.4166 Y43.3897\nG1 X197.86 Y44.1402\nG1 X197.2325 Y44.8325\nG1 X196.5401 Y45.46\nG1 X195.7896 Y46.0166\nG1 X194.9882 Y46.4969\nG1 X194.1436 Y46.8964\nG1 X193.2639 Y47.2112\nG1 X192.3575 Y47.4382\nG1 X191.4332 Y47.5753\nG1 X190.4222 Y47.625\nG1 X12.6221\nG1 Z-13.8887 F250\nG1 X11.1436 Y47.6976 F1000\nG1 X9.6022 Y47.9263\nG1 X8.0906 Y48.3049\nG1 X6.6235 Y48.8299\nG1 X5.2148 Y49.4961\nG1 X3.8782 Y50.2972\nG1 X2.6266 Y51.2255\nG1 X1.472 Y52.272\nG1 X0.4255 Y53.4266\nG1 X-0.5028 Y54.6782\nG1 X-1.3039 Y56.0148\nG1 X-1.9701 Y57.4234\nG1 X-2.4951 Y58.8906\nG1 X-2.8737 Y60.4022\nG1 X-3.1024 Y61.9436\nG1 X-3.175 Y63.4221\nG1 Y177.8779\nG1 X-3.1024 Y179.3564\nG1 X-2.8737 Y180.8978\nG1 X-2.4951 Y182.4094\nG1 X-1.9701 Y183.8766\nG1 X-1.3039 Y185.2853\nG1 X-0.5028 Y186.6218\nG1 X0.4255 Y187.8734\nG1 X1.472 Y189.028\nG1 X2.6266 Y190.0745\nG1 X3.8782 Y191.0028\nG1 X5.2148 Y191.8039\nG1 X6.6235 Y192.4701\nG1 X8.0906 Y192.9951\nG1 X9.6022 Y193.3737\nG1 X11.1436 Y193.6024\nG1 X12.6221 Y193.675\nG1 X190.4222\nG1 X191.4332 Y193.7247\nG1 X192.3575 Y193.8618\nG1 X193.2639 Y194.0888\nG1 X194.1436 Y194.4036\nG1 X194.9882 Y194.8031\nG1 X195.7896 Y195.2834\nG1 X196.5401 Y195.84\nG1 X197.2325 Y196.4675\nG1 X197.86 Y197.1598\nG1 X198.4166 Y197.9103\nG1 X198.8969 Y198.7117\nG1 X199.2964 Y199.5564\nG1 X199.6112 Y200.4362\nG1 X199.8382 Y201.3426\nG1 X199.9753 Y202.2668\nG1 X200.025 Y203.278\nG1 Y228.6779\nG1 X200.0976 Y230.1564\nG1 X200.3263 Y231.6978\nG1 X200.7049 Y233.2094\nG1 X201.2299 Y234.6766\nG1 X201.8961 Y236.0852\nG1 X202.6972 Y237.4218\nG1 X203.6255 Y238.6734\nG1 X204.672 Y239.828\nG1 X205.8266 Y240.8745\nG1 X207.0782 Y241.8028\nG1 X208.4148 Y242.6039\nG1 X209.8234 Y243.2701\nG1 X211.2906 Y243.7951\nG1 X212.8022 Y244.1737\nG1 X214.3436 Y244.4024\nG1 X215.8221 Y244.475\nG1 X257.175\nG1 Y-3.175\nG1 X215.8221\nG1 X214.3436 Y-3.1024\nG1 X212.8022 Y-2.8737\nG1 X211.2906 Y-2.4951\nG1 X209.8234 Y-1.9701\nG1 X208.4148 Y-1.3039\nG1 X207.0782 Y-0.5028\nG1 X205.8266 Y0.4255\nG1 X204.672 Y1.472\nG1 X203.6255 Y2.6266\nG1 X202.6972 Y3.8782\nG1 X201.8961 Y5.2148\nG1 X201.2299 Y6.6234\nG1 X200.7049 Y8.0906\nG1 X200.3263 Y9.6022\nG1 X200.0976 Y11.1436\nG1 X200.025 Y12.6221\nG1 Y38.022\nG1 X199.9753 Y39.0332\nG1 X199.8382 Y39.9574\nG1 X199.6112 Y40.8638\nG1 X199.2964 Y41.7436\nG1 X198.8969 Y42.5883\nG1 X198.4166 Y43.3897\nG1 X197.86 Y44.1402\nG1 X197.2325 Y44.8325\nG1 X196.5401 Y45.46\nG1 X195.7896 Y46.0166\nG1 X194.9882 Y46.4969\nG1 X194.1436 Y46.8964\nG1 X193.2639 Y47.2112\nG1 X192.3575 Y47.4382\nG1 X191.4332 Y47.5753\nG1 X190.4222 Y47.625\nG1 X12.6221\nG0 Z1.0 F300\nG0 X132.675 Y193.675 F6000\nG1 Z-15.179 F250\nG1 X190.4222 F1000\nG1 X191.4332 Y193.7247\nG1 X192.3575 Y193.8618\nG1 X193.2639 Y194.0888\nG1 X194.1436 Y194.4036\nG1 X194.9882 Y194.8031\nG1 X195.7896 Y195.2834\nG1 X196.5401 Y195.84\nG1 X197.2325 Y196.4675\nG1 X197.86 Y197.1598\nG1 X198.4166 Y197.9103\nG1 X198.8969 Y198.7117\nG1 X199.2964 Y199.5564\nG1 X199.6112 Y200.4362\nG1 X199.8382 Y201.3426\nG1 X199.9753 Y202.2668\nG1 X200.025 Y203.278\nG1 Y228.6779\nG1 X200.0976 Y230.1564\nG1 X200.3263 Y231.6978\nG1 X200.7049 Y233.2094\nG1 X201.2299 Y234.6766\nG1 X201.8961 Y236.0852\nG1 X202.6972 Y237.4218\nG1 X203.6255 Y238.6734\nG1 X204.672 Y239.828\nG1 X205.8266 Y240.8745\nG1 X207.0782 Y241.8028\nG1 X208.4148 Y242.6039\nG1 X209.8234 Y243.2701\nG1 X211.2906 Y243.7951\nG1 X212.8022 Y244.1737\nG1 X214.3436 Y244.4024\nG1 X215.8221 Y244.475\nG1 X257.175\nG1 Y126.325\nG0 Z1.0 F300\nG0 X132.675 Y193.675 F6000\nG1 Z-17.1145 F250\nG1 X190.4222 F1000\nG1 X191.4332 Y193.7247\nG1 X192.3575 Y193.8618\nG1 X193.2639 Y194.0888\nG1 X194.1436 Y194.4036\nG1 X194.9882 Y194.8031\nG1 X195.7896 Y195.2834\nG1 X196.5401 Y195.84\nG1 X197.2325 Y196.4675\nG1 X197.86 Y197.1598\nG1 X198.4166 Y197.9103\nG1 X198.8969 Y198.7117\nG1 X199.2964 Y199.5564\nG1 X199.6112 Y200.4362\nG1 X199.8382 Y201.3426\nG1 X199.9753 Y202.2668\nG1 X200.025 Y203.278\nG1 Y228.6779\nG1 X200.0976 Y230.1564\nG1 X200.3263 Y231.6978\nG1 X200.7049 Y233.2094\nG1 X201.2299 Y234.6766\nG1 X201.8961 Y236.0852\nG1 X202.6972 Y237.4218\nG1 X203.6255 Y238.6734\nG1 X204.672 Y239.828\nG1 X205.8266 Y240.8745\nG1 X207.0782 Y241.8028\nG1 X208.4148 Y242.6039\nG1 X209.8234 Y243.2701\nG1 X211.2906 Y243.7951\nG1 X212.8022 Y244.1737\nG1 X214.3436 Y244.4024\nG1 X215.8221 Y244.475\nG1 X257.175\nG1 Y126.325\nG0 Z1.0 F300\nG0 X132.675 Y193.675 F6000\nG1 Z-19.05 F250\nG1 X190.4222 F1000\nG1 X191.4332 Y193.7247\nG1 X192.3575 Y193.8618\nG1 X193.2639 Y194.0888\nG1 X194.1436 Y194.4036\nG1 X194.9882 Y194.8031\nG1 X195.7896 Y195.2834\nG1 X196.5401 Y195.84\nG1 X197.2325 Y196.4675\nG1 X197.86 Y197.1598\nG1 X198.4166 Y197.9103\nG1 X198.8969 Y198.7117\nG1 X199.2964 Y199.5564\nG1 X199.6112 Y200.4362\nG1 X199.8382 Y201.3426\nG1 X199.9753 Y202.2668\nG1 X200.025 Y203.278\nG1 Y228.6779\nG1 X200.0976 Y230.1564\nG1 X200.3263 Y231.6978\nG1 X200.7049 Y233.2094\nG1 X201.2299 Y234.6766\nG1 X201.8961 Y236.0852\nG1 X202.6972 Y237.4218\nG1 X203.6255 Y238.6734\nG1 X204.672 Y239.828\nG1 X205.8266 Y240.8745\nG1 X207.0782 Y241.8028\nG1 X208.4148 Y242.6039\nG1 X209.8234 Y243.2701\nG1 X211.2906 Y243.7951\nG1 X212.8022 Y244.1737\nG1 X214.3436 Y244.4024\nG1 X215.8221 Y244.475\nG1 X257.175\nG1 Y126.325\nG0 Z1.0 F300\nG0 X132.675 Y47.625 F6000\nG1 Z-15.179 F300\nG1 X190.4222 F1000\nG1 X191.4332 Y47.5753\nG1 X192.3575 Y47.4382\nG1 X193.2639 Y47.2112\nG1 X194.1436 Y46.8964\nG1 X194.9882 Y46.4969\nG1 X195.7896 Y46.0166\nG1 X196.5401 Y45.46\nG1 X197.2325 Y44.8325\nG1 X197.86 Y44.1402\nG1 X198.4166 Y43.3897\nG1 X198.8969 Y42.5883\nG1 X199.2964 Y41.7436\nG1 X199.6112 Y40.8638\nG1 X199.8382 Y39.9574\nG1 X199.9753 Y39.0332\nG1 X200.025 Y38.022\nG1 Y12.6221\nG1 X200.0976 Y11.1436\nG1 X200.3263 Y9.6022\nG1 X200.7049 Y8.0906\nG1 X201.2299 Y6.6234\nG1 X201.8961 Y5.2148\nG1 X202.6972 Y3.8782\nG1 X203.6255 Y2.6266\nG1 X204.672 Y1.472\nG1 X205.8266 Y0.4255\nG1 X207.0782 Y-0.5028\nG1 X208.4148 Y-1.3039\nG1 X209.8234 Y-1.9701\nG1 X211.2906 Y-2.4951\nG1 X212.8022 Y-2.8737\nG1 X214.3436 Y-3.1024\nG1 X215.8221 Y-3.175\nG1 X257.175\nG1 Y114.975\nG0 Z1.0 F300\nG0 X132.675 Y47.625 F6000\nG1 Z-17.1145 F250\nG1 X190.4222 F1000\nG1 X191.4332 Y47.5753\nG1 X192.3575 Y47.4382\nG1 X193.2639 Y47.2112\nG1 X194.1436 Y46.8964\nG1 X194.9882 Y46.4969\nG1 X195.7896 Y46.0166\nG1 X196.5401 Y45.46\nG1 X197.2325 Y44.8325\nG1 X197.86 Y44.1402\nG1 X198.4166 Y43.3897\nG1 X198.8969 Y42.5883\nG1 X199.2964 Y41.7436\nG1 X199.6112 Y40.8638\nG1 X199.8382 Y39.9574\nG1 X199.9753 Y39.0332\nG1 X200.025 Y38.022\nG1 Y12.6221\nG1 X200.0976 Y11.1436\nG1 X200.3263 Y9.6022\nG1 X200.7049 Y8.0906\nG1 X201.2299 Y6.6234\nG1 X201.8961 Y5.2148\nG1 X202.6972 Y3.8782\nG1 X203.6255 Y2.6266\nG1 X204.672 Y1.472\nG1 X205.8266 Y0.4255\nG1 X207.0782 Y-0.5028\nG1 X208.4148 Y-1.3039\nG1 X209.8234 Y-1.9701\nG1 X211.2906 Y-2.4951\nG1 X212.8022 Y-2.8737\nG1 X214.3436 Y-3.1024\nG1 X215.8221 Y-3.175\nG1 X257.175\nG1 Y114.975\nG0 Z1.0 F300\nG0 X132.675 Y47.625 F6000\nG1 Z-19.05 F250\nG1 X190.4222 F1000\nG1 X191.4332 Y47.5753\nG1 X192.3575 Y47.4382\nG1 X193.2639 Y47.2112\nG1 X194.1436 Y46.8964\nG1 X194.9882 Y46.4969\nG1 X195.7896 Y46.0166\nG1 X196.5401 Y45.46\nG1 X197.2325 Y44.8325\nG1 X197.86 Y44.1402\nG1 X198.4166 Y43.3897\nG1 X198.8969 Y42.5883\nG1 X199.2964 Y41.7436\nG1 X199.6112 Y40.8638\nG1 X199.8382 Y39.9574\nG1 X199.9753 Y39.0332\nG1 X200.025 Y38.022\nG1 Y12.6221\nG1 X200.0976 Y11.1436\nG1 X200.3263 Y9.6022\nG1 X200.7049 Y8.0906\nG1 X201.2299 Y6.6234\nG1 X201.8961 Y5.2148\nG1 X202.6972 Y3.8782\nG1 X203.6255 Y2.6266\nG1 X204.672 Y1.472\nG1 X205.8266 Y0.4255\nG1 X207.0782 Y-0.5028\nG1 X208.4148 Y-1.3039\nG1 X209.8234 Y-1.9701\nG1 X211.2906 Y-2.4951\nG1 X212.8022 Y-2.8737\nG1 X214.3436 Y-3.1024\nG1 X215.8221 Y-3.175\nG1 X257.175\nG1 Y114.975\nG0 Z1.0 F300\nG0 X121.325 Y193.675 F6000\nG1 Z-15.179 F300\nG1 X12.6221 F1000\nG1 X11.1436 Y193.6024\nG1 X9.6022 Y193.3737\nG1 X8.0906 Y192.9951\nG1 X6.6235 Y192.4701\nG1 X5.2148 Y191.8039\nG1 X3.8782 Y191.0028\nG1 X2.6266 Y190.0745\nG1 X1.472 Y189.028\nG1 X0.4255 Y187.8734\nG1 X-0.5028 Y186.6218\nG1 X-1.3039 Y185.2853\nG1 X-1.9701 Y183.8766\nG1 X-2.4951 Y182.4094\nG1 X-2.8737 Y180.8978\nG1 X-3.1024 Y179.3564\nG1 X-3.175 Y177.8779\nG1 Y126.325\nG0 Z1.0 F300\nG0 X121.325 Y193.675 F6000\nG1 Z-17.1145 F250\nG1 X12.6221 F1000\nG1 X11.1436 Y193.6024\nG1 X9.6022 Y193.3737\nG1 X8.0906 Y192.9951\nG1 X6.6235 Y192.4701\nG1 X5.2148 Y191.8039\nG1 X3.8782 Y191.0028\nG1 X2.6266 Y190.0745\nG1 X1.472 Y189.028\nG1 X0.4255 Y187.8734\nG1 X-0.5028 Y186.6218\nG1 X-1.3039 Y185.2853\nG1 X-1.9701 Y183.8766\nG1 X-2.4951 Y182.4094\nG1 X-2.8737 Y180.8978\nG1 X-3.1024 Y179.3564\nG1 X-3.175 Y177.8779\nG1 Y126.325\nG0 Z1.0 F300\nG0 X121.325 Y193.675 F6000\nG1 Z-19.05 F250\nG1 X12.6221 F1000\nG1 X11.1436 Y193.6024\nG1 X9.6022 Y193.3737\nG1 X8.0906 Y192.9951\nG1 X6.6235 Y192.4701\nG1 X5.2148 Y191.8039\nG1 X3.8782 Y191.0028\nG1 X2.6266 Y190.0745\nG1 X1.472 Y189.028\nG1 X0.4255 Y187.8734\nG1 X-0.5028 Y186.6218\nG1 X-1.3039 Y185.2853\nG1 X-1.9701 Y183.8766\nG1 X-2.4951 Y182.4094\nG1 X-2.8737 Y180.8978\nG1 X-3.1024 Y179.3564\nG1 X-3.175 Y177.8779\nG1 Y126.325\nG0 Z1.0 F300\nG0 X121.325 Y47.625 F6000\nG1 Z-15.179 F300\nG1 X12.6221 F1000\nG1 X11.1436 Y47.6976\nG1 X9.6022 Y47.9263\nG1 X8.0906 Y48.3049\nG1 X6.6235 Y48.8299\nG1 X5.2148 Y49.4961\nG1 X3.8782 Y50.2972\nG1 X2.6266 Y51.2255\nG1 X1.472 Y52.272\nG1 X0.4255 Y53.4266\nG1 X-0.5028 Y54.6782\nG1 X-1.3039 Y56.0148\nG1 X-1.9701 Y57.4234\nG1 X-2.4951 Y58.8906\nG1 X-2.8737 Y60.4022\nG1 X-3.1024 Y61.9436\nG1 X-3.175 Y63.4221\nG1 Y114.975\nG0 Z1.0 F300\nG0 X121.325 Y47.625 F6000\nG1 Z-17.1145 F250\nG1 X12.6221 F1000\nG1 X11.1436 Y47.6976\nG1 X9.6022 Y47.9263\nG1 X8.0906 Y48.3049\nG1 X6.6235 Y48.8299\nG1 X5.2148 Y49.4961\nG1 X3.8782 Y50.2972\nG1 X2.6266 Y51.2255\nG1 X1.472 Y52.272\nG1 X0.4255 Y53.4266\nG1 X-0.5028 Y54.6782\nG1 X-1.3039 Y56.0148\nG1 X-1.9701 Y57.4234\nG1 X-2.4951 Y58.8906\nG1 X-2.8737 Y60.4022\nG1 X-3.1024 Y61.9436\nG1 X-3.175 Y63.4221\nG1 Y114.975\nG0 Z1.0 F300\nG0 X121.325 Y47.625 F6000\nG1 Z-19.05 F250\nG1 X12.6221 F1000\nG1 X11.1436 Y47.6976\nG1 X9.6022 Y47.9263\nG1 X8.0906 Y48.3049\nG1 X6.6235 Y48.8299\nG1 X5.2148 Y49.4961\nG1 X3.8782 Y50.2972\nG1 X2.6266 Y51.2255\nG1 X1.472 Y52.272\nG1 X0.4255 Y53.4266\nG1 X-0.5028 Y54.6782\nG1 X-1.3039 Y56.0148\nG1 X-1.9701 Y57.4234\nG1 X-2.4951 Y58.8906\nG1 X-2.8737 Y60.4022\nG1 X-3.1024 Y61.9436\nG1 X-3.175 Y63.4221\nG1 Y114.975\nG0 Z1.0 F300\nM30"
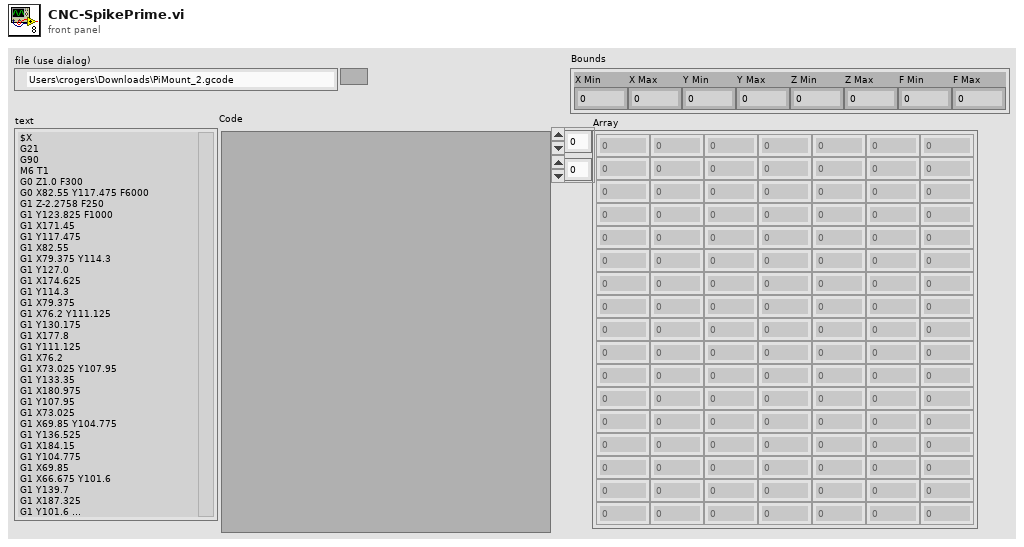
[diagram p1: front panel]
types:
  T1 = cluster{"X Min":dbl, "X Max":dbl, "Y Min":dbl, "Y Max":dbl, "Z Min":dbl, "Z Max":dbl, "F Min":dbl, "F Max":dbl}
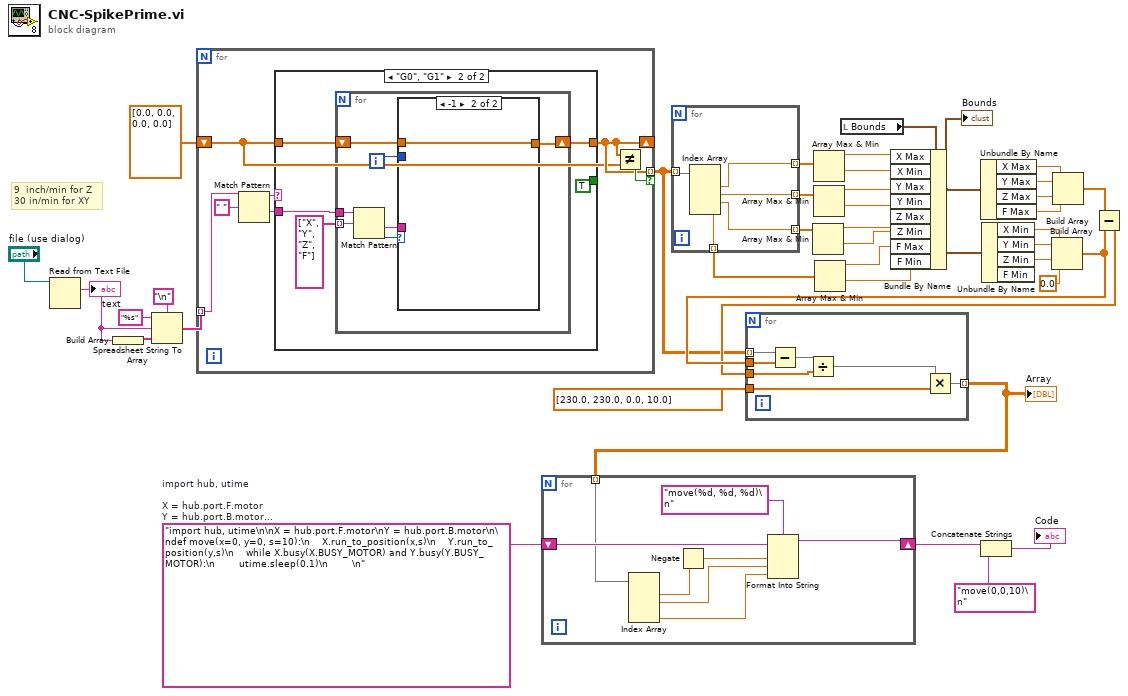
[diagram p0: block diagram]
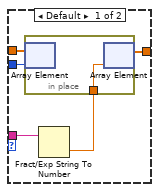
[diagram p3: hidden frame]
diagram:
  w9 = "import hub, utime\n\nX = hub.port.F.motor\nY = hub.port.B.motor\n\ndef move(x=0, y=0, s=10):\n    X.run_to_position(x,s)\n    Y.run_to_position(y,s)\n    while X.busy(X.BUSY_MOTOR) and Y.busy(Y.BUSY_MOTOR):\n        utime.sleep(0.1)\n        \n"  # import hub, utime  X = hub.port.F.motor Y = hub.port.B.motor  def move(x=0, y=0, s=10):     X.run_to_position(x,s)     Y.run_to_position(y,s)     while X.busy(X.BUSY_MOTOR) and Y.busy(Y.BUSY_MOTOR):         utime.sleep(0.1)
  # "9  inch/min for Z\n30 in/min for XY"
  n1 = Read from Text File(file (use dialog)="file (use dialog)") -> (text=w1:string)  [unwired: 3 in, 3 out]
  "text" <- w1
  n2 = Build Array(w1) -> (w38:string[])
  n3 = Spreadsheet String To Array(delimiter (Tab)="\n", format string="%s", spreadsheet string=w1, array type (2D Dbl)=w38) -> (array=w35:string[])
  n4 = for {
    tunnel: w35 -> [w46] mode=indexing
    shift-right: [w41] -> _
    shift-left: dbl[] [0.0, 0.0, 0.0, 0.0] -> [w40]
    tunnel: [w41] -> w8 mode=indexing if=w42
    n5 = Match Pattern(string=w46, regular expression=" ") -> (before substring=w44:string, after substring=w43:string)  [unwired: 1 in, 2 out]
    n6 = case shown="\"G0\", \"G1\"" w44 {
      tunnel: w40 -> [w47 w51]
      tunnel: [w47 w50] -> w41
      tunnel: w43 -> [_ w49]
      tunnel: [_ TRUE] -> _
      frame Default {
      }
      frame "G0", "G1" {
        n7 = for {
          tunnel: string[] ["X", "Y", "Z", "F"] -> [w59] mode=indexing
          shift-right: [w54] -> w50
          shift-left: w51 -> [w57]
          tunnel: w49 -> [w53]
          i -> [w56]
          n8 = Match Pattern(string=w53, regular expression=w59) -> (after substring=w55:string, offset past match=w58:i32)  [unwired: 1 in, 2 out]
          n9 = case shown="-1" w58 {
            tunnel: w57 -> [w64 w66]
            tunnel: w56 -> [w63 _]
            tunnel: w55 -> [w62 _]
            tunnel: [w60 w66] -> w54
            frame Default {
              n10 = Fract/Exp String To Number(string=w62) -> (number=w61:dbl)  [unwired: 3 in, 1 out]
              n11 = in-place {
                in-place-border: w61 -> [w65]
                n12 = in-place-array #1(w64, w63) -> ()  [unwired: 1 out]
                n13 = in-place-array #1(w65) -> (w60:dbl[])  [unwired: 1 out]
              }
            }
            frame -1 {
            }
          }
        }
      }
    }
    n14 = Not Equal?(x=w41, y=w40) -> (x != y?=w42:bool)
  }
  n15 = for {
    tunnel: [w71] -> w33 mode=indexing
    tunnel: [w70] -> w32 mode=indexing
    tunnel: [w69] -> w31 mode=indexing
    tunnel: w8 -> [w68] mode=indexing
    tunnel: [w67] -> w13 mode=indexing
    n16 = Index Array(array=w68) -> (element #1=w71:dbl, element #2=w70:dbl, element #3=w69:dbl, element #4=w67:dbl)  [unwired: 4 in]
  }
  n17 = Array Max & Min(array=w31) -> (max value=w28:dbl, min value=w29:dbl)  [unwired: 2 out]
  n18 = Array Max & Min(array=w33) -> (max value=w24:dbl, min value=w25:dbl)  [unwired: 2 out]
  n19 = Array Max & Min(array=w32) -> (max value=w26:dbl, min value=w27:dbl)  [unwired: 2 out]
  n20 = Array Max & Min(array=w13) -> (max value=w12:dbl, min value=w11:dbl)  [unwired: 2 out]
  n21 = local read "Bounds"() -> (w30:T1)
  n22 = Bundle By Name(cluster=w30, "X Max"=w24, "X Min"=w25, "Y Max"=w26, "Y Min"=w27, "Z Max"=w28, "Z Min"=w29, "F Max"=w12, "F Min"=w11) -> (w17:T1)
  "Bounds" <- w17
  n23 = Unbundle By Name(w17) -> ("X Max"=w18:dbl, "Y Max"=w19:dbl, "Z Max"=w20:dbl, "F Max"=w5:dbl)
  n24 = Unbundle By Name(w17) -> ("X Min"=w23:dbl, "Y Min"=w22:dbl, "Z Min"=w21:dbl)  [unwired: 1 out]
  n25 = Build Array(w23, w22, w21, 0.0) -> (w15:dbl[])
  n26 = Build Array(w18, w19, w20, w5) -> (w16:dbl[])
  n27 = Subtract(x=w16, y=w15) -> (x-y=w14:dbl[])
  n28 = for {
    tunnel: w8 -> [w78] mode=indexing
    tunnel: w15 -> [w77]
    tunnel: w14 -> [w75]
    tunnel: dbl[] [230.0, 230.0, 0.0, 10.0] -> [w73]
    tunnel: [w72] -> w7 mode=indexing
    n29 = Subtract(x=w78, y=w77) -> (x-y=w76:dbl[])
    n30 = Divide(x=w76, y=w75) -> (x/y=w74:dbl[])
    n31 = Multiply(x=w74, y=w73) -> (x*y=w72:dbl[])
  }
  "Array" <- w7
  n32 = for {
    shift-right: [w84] -> w3
    shift-left: w9 -> [w85]
    tunnel: w7 -> [w83] mode=indexing
    n33 = Index Array(array=w83) -> (element #1=w82:dbl, element #2=w80:dbl, element #4=w81:dbl)  [unwired: 4 in, 1 out]
    n34 = Negate(x=w82) -> (-x=w79:dbl)
    n35 = Format Into String(format string="move(%d, %d, %d)\n", initial string=w85, w79, w80, w81) -> (resulting string=w84:string)  [unwired: 1 in, 1 out]
  }
  n36 = Concatenate Strings(w3, "move(0,0,10)\n" ("format string")) -> (→"Code":string)
